vi "TRIQUI.vi"() -> ()   [LabVIEW 2020]
uses:
  Control 2.ctl
panel:
  in  "Nueva Partida":T1
  in  "Salir del Juego":bool
  out "Turno":string
  in  "Ring 9":u16(ring)
  in  "Ring 8":u16(ring)
  in  "Ring 7":u16(ring)
  in  "Ring 6":u16(ring)
  in  "Ring 5":u16(ring)
  in  "Ring 4":u16(ring)
  in  "Ring 3":u16(ring)
  in  "Ring 2":u16(ring)
  in  "Ring":u16(ring)
  # "TRIQUI"
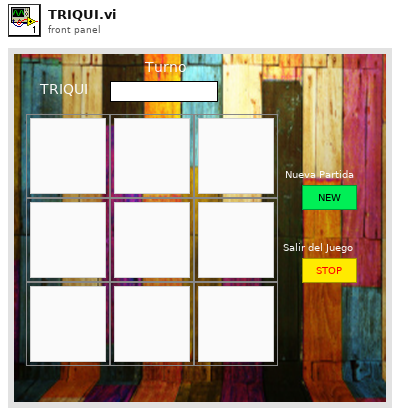
[diagram p1: front panel]
types:
  T1 = typedef "Control 2.ctl" = bool
  T2 = typedef "Symbol.ctl" = u16
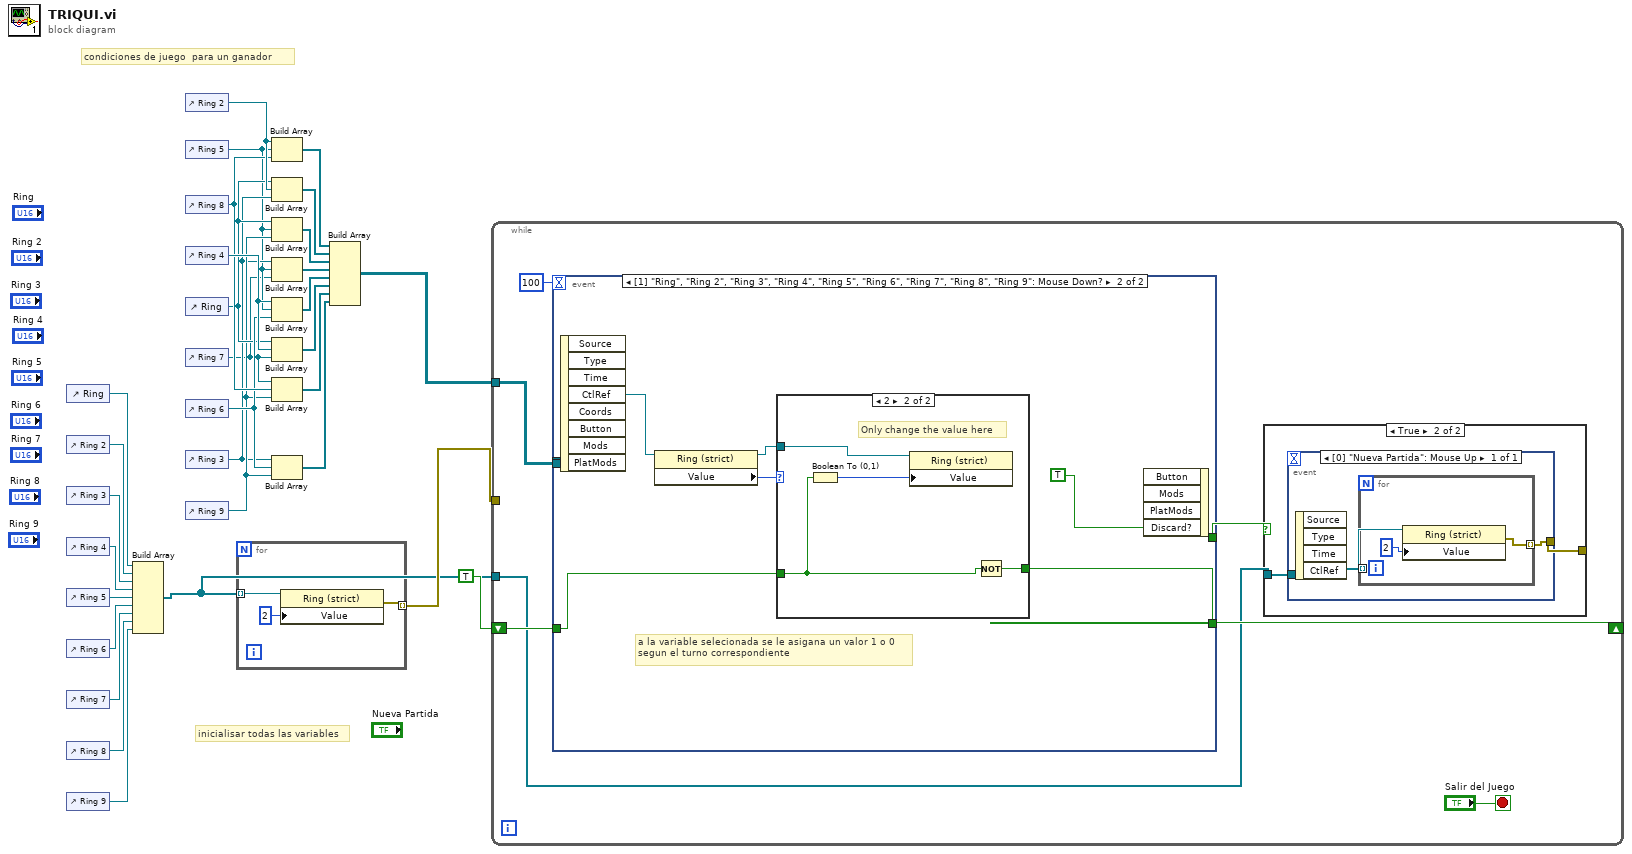
[diagram p0: block diagram]
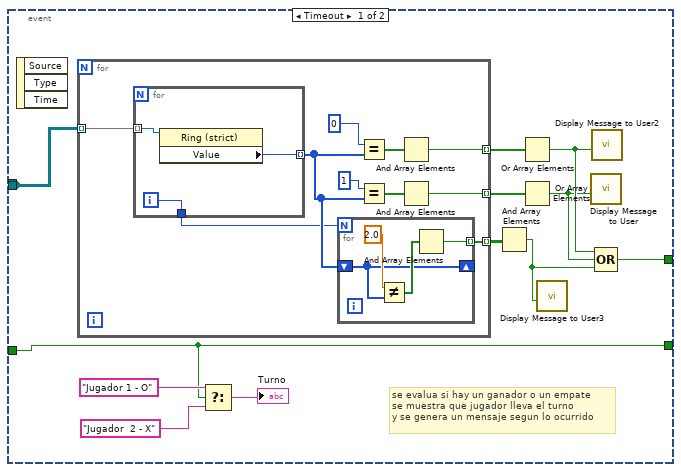
[diagram p3: hidden frame]
diagram:
  # "condiciones de juego  para un ganador"
  # "inicialisar todas las variables"
  n1 = control-ref of="Ring"() -> (w30:refnum<vi>)
  n2 = control-ref of="Ring 2"() -> (w29:refnum<vi>)
  n3 = control-ref of="Ring 3"() -> (w28:refnum<vi>)
  n4 = control-ref of="Ring 4"() -> (w27:refnum<vi>)
  n5 = control-ref of="Ring 5"() -> (w26:refnum<vi>)
  n6 = control-ref of="Ring 6"() -> (w5:refnum<vi>)
  n7 = control-ref of="Ring 7"() -> (w4:refnum<vi>)
  n8 = control-ref of="Ring 8"() -> (w3:refnum<vi>)
  n9 = control-ref of="Ring 9"() -> (w2:refnum<vi>)
  n10 = Build Array(w30, w29, w28, w27, w26, w5, w4, w3, w2) -> (w1:refnum<vi>[])
  n11 = control-ref of="Ring 2"() -> (w24:refnum<vi>)
  n12 = control-ref of="Ring 5"() -> (w18:refnum<vi>)
  n13 = control-ref of="Ring 8"() -> (w23:refnum<vi>)
  n14 = control-ref of="Ring 4"() -> (w25:refnum<vi>)
  n15 = control-ref of="Ring"() -> (w21:refnum<vi>)
  n16 = control-ref of="Ring 7"() -> (w17:refnum<vi>)
  n17 = control-ref of="Ring 6"() -> (w22:refnum<vi>)
  n18 = control-ref of="Ring 3"() -> (w19:refnum<vi>)
  n19 = control-ref of="Ring 9"() -> (w20:refnum<vi>)
  n20 = for {
    tunnel: w1 -> [w33] mode=indexing
    tunnel: [w31] -> w6 mode=indexing
    n21 = property class="Ring (strict)"(reference=w33, "Value"=u16 2) -> (error out=w31:errorcluster)  [unwired: 1 in, 1 out]
  }
  n22 = Build Array(w24, w18, w23) -> (w16:refnum<vi>[])
  n23 = Build Array(w21, w24, w19) -> (w15:refnum<vi>[])
  n24 = Build Array(w21, w18, w20) -> (w14:refnum<vi>[])
  n25 = Build Array(w19, w18, w17) -> (w13:refnum<vi>[])
  n26 = Build Array(w25, w18, w22) -> (w12:refnum<vi>[])
  n27 = Build Array(w21, w25, w17) -> (w11:refnum<vi>[])
  n28 = Build Array(w17, w23, w20) -> (w10:refnum<vi>[])
  n29 = Build Array(w19, w22, w20) -> (w9:refnum<vi>[])
  n30 = Build Array(w16, w15, w14, w13, w12, w11, w10, w9) -> (w8:refnum<vi>[][])
  n31 = while {
    tunnel: w8 -> [w40]
    shift-right: [w38] -> _
    shift-left: TRUE -> [w39]
    tunnel: w6 -> [_]
    tunnel: w1 -> [w34]
    stop <- "Salir del Juego" stop-if-true
    n32 = event shown="[1] \"Ring\", \"Ring 2\", \"Ring 3\", \"Ring 4\", \"Ring 5\", \"Ring 6\", \"Ring 7\", \"Ring 8\", \"Ring 9\": Mouse Down?" {
      selector: _ -> [_ _]
      dyn-events: _ -> [_ _]
      timeout: 100 -> [_ _]
      tunnel: [w53 _] -> _
      tunnel: w40 -> [w53 _]
      tunnel: w39 -> [w54 w79]
      tunnel: [w54 w78] -> w38
      tunnel: [w48 _] -> w35
      event Timeout {
        # "se evalua si hay un ganador o un empate \nse muestra que jugador lleva el turno \ny se genera un mensaje segun lo ocurrido"
        n33 = event-data() -> ()  [unwired: 1 in, 3 out]
        n34 = for {
          tunnel: [w67] -> w55 mode=indexing
          tunnel: [w66] -> w56 mode=indexing
          tunnel: w53 -> [w65] mode=indexing
          tunnel: [w61] -> w52 mode=indexing
          n35 = for {
            tunnel: [w76] -> w62 mode=indexing
            tunnel: w65 -> [w75] mode=indexing
            tunnel: [w74] -> w60
            i -> [w74]
            n36 = property class="Ring (strict)"(reference=w75) -> ("Value"=w76:T2)  [unwired: 1 in, 2 out]
          }
          n37 = for {
            N: w60 -> [_]
            shift-right: [w71] -> _
            shift-left: w62 -> [w71]
            tunnel: [w70] -> w61 mode=indexing
            n38 = Not Equal?(x=2.0, y=w71) -> (x != y?=w73:bool[])
            n39 = And Array Elements(Boolean array=w73) -> (logical AND=w70:bool)
          }
          n40 = Equal?(x=0, y=w62) -> (x = y?=w69:bool[])
          n41 = Equal?(x=1, y=w62) -> (x = y?=w68:bool[])
          n42 = And Array Elements(Boolean array=w69) -> (logical AND=w66:bool)
          n43 = And Array Elements(Boolean array=w68) -> (logical AND=w67:bool)
        }
        n44 = Select(t="Jugador 1 - O", s=w54, f="Jugador  2 - X") -> (s? t:f=→"Turno":string)
        n45 = And Array Elements(Boolean array=w52) -> (logical AND=w49:bool)
        n46 = Or Array Elements(Boolean array=w56) -> (logical OR=w51:bool)
        n47 = Or Array Elements(Boolean array=w55) -> (logical OR=w50:bool)
        n48 = call "Display Message to User3"("Enable"=w49) -> ()  [unwired: 9 in, 2 out]
        n49 = call "Display Message to User"("Enable"=w50) -> ()  [unwired: 9 in, 2 out]
        n50 = call "Display Message to User2"("Enable"=w51) -> ()  [unwired: 9 in, 2 out]
        n51 = Compound Arithmetic op=OR(w51, w50, w49) -> (w48:bool)
      }
      event "Ring", "Ring 2", "Ring 3", "Ring 4", "Ring 5", "Ring 6", "Ring 7", "Ring 8", "Ring 9": Mouse Down? {
        # "a la variable selecionada se le asigana un valor 1 o 0 \nsegun el turno correspondiente"
        n52 = event-data() -> ("CtlRef"=w77:refnum<vi>)  [unwired: 1 in, 7 out]
        n53 = property class="Ring (strict)"(reference=w77) -> (reference out=w81:refnum<vi>, "Value"=w82:T2)  [unwired: 1 in, 1 out]
        n54 = case shown="2" w82 {
          tunnel: [w83 w87] -> w78
          tunnel: w81 -> [_ w86]
          tunnel: w79 -> [w83 w84]
          frame Default {
            # "DO not touch the values here"
          }
          frame 2 {
            # "Only change the value here"
            n55 = Boolean To (0,1)(Boolean=w84) -> (0, 1=w85:i16)
            n56 = property class="Ring (strict)"(reference=w86, "Value"=w85) -> ()  [unwired: 1 in, 2 out]
            n57 = Not(x=w84) -> (.not. x?=w87:bool)
          }
        }
        n58 = event-data("Discard?"=TRUE) -> ()  [unwired: 4 in, 1 out]
      }
    }
    n59 = case shown="True" w35 {
      tunnel: w34 -> [_ w42]
      tunnel: [_ w41] -> _
      frame False {
      }
      frame True {
        n60 = event shown="[0] \"Nueva Partida\": Mouse Up" {
          selector: _ -> [_]
          dyn-events: _ -> [_]
          timeout: _ -> [_]
          tunnel: w42 -> [w44]
          tunnel: [w43] -> w41
          event Mouse Up {
            n61 = event-data() -> ()  [unwired: 1 in, 4 out]
            n62 = for {
              tunnel: w44 -> [w46] mode=indexing
              tunnel: [w45] -> w43 mode=indexing
              n63 = property class="Ring (strict)"(reference=w46, "Value"=u16 2) -> (error out=w45:errorcluster)  [unwired: 1 in, 1 out]
            }
          }
        }
      }
    }
  }
